vi "Application_WaitMsInError.vi"(10 "Errorin":errorcluster, 11 "ms":u32) -> (2 "Errorout":errorcluster)   [LabVIEW 2016]
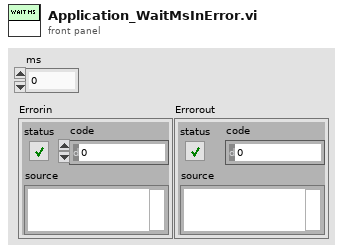
[diagram p1: front panel]
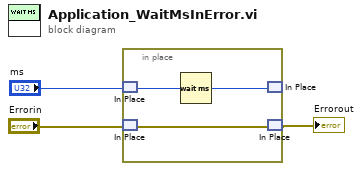
[diagram p0: block diagram]
diagram:
  n1 = in-place {
    n2 = in-place-match #1("ms") -> (w5:u32)
    n3 = in-place-match #2("Errorin") -> (w6:errorcluster)
    n4 = Wait (ms)(milliseconds to wait=w5) -> (millisecond timer value=w4:u32)
    n5 = in-place-match #1(w4) -> ()  [unwired: 1 out]
    n6 = in-place-match #2(w6) -> (→"Errorout":errorcluster)
  }
